vi "Python toolkit.vi"(8 "error in (no error)":errorcluster) -> (0 "error out":errorcluster)   [LabVIEW 2018]
uses:
  Python Toolkit/Python Toolkit.lvclass
  Python Toolkit/Python Toolkit.lvclass/Python Toolkit.ctl
  <vilib>/addons/_JKI Toolkits/Caraya/classes/Assert/Assert Equal Value_Variant.vi
  <vilib>/addons/_JKI Toolkits/Caraya/classes/Assert/Assert Not Error.vi
  <vilib>/addons/_JKI Toolkits/Caraya/classes/Test/Test.lvclass
  <vilib>/addons/_JKI Toolkits/Caraya/classes/Assert/Assert.lvclass
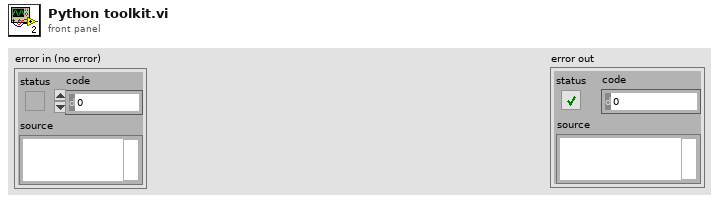
[diagram p1: front panel]
types:
  T1 = cluster{"CCD":string, "S4GUI":string, "S4ICS":string, "TCS":string, "FOCUSER":string, "WSTATION":string, "GENERAL KW":string}
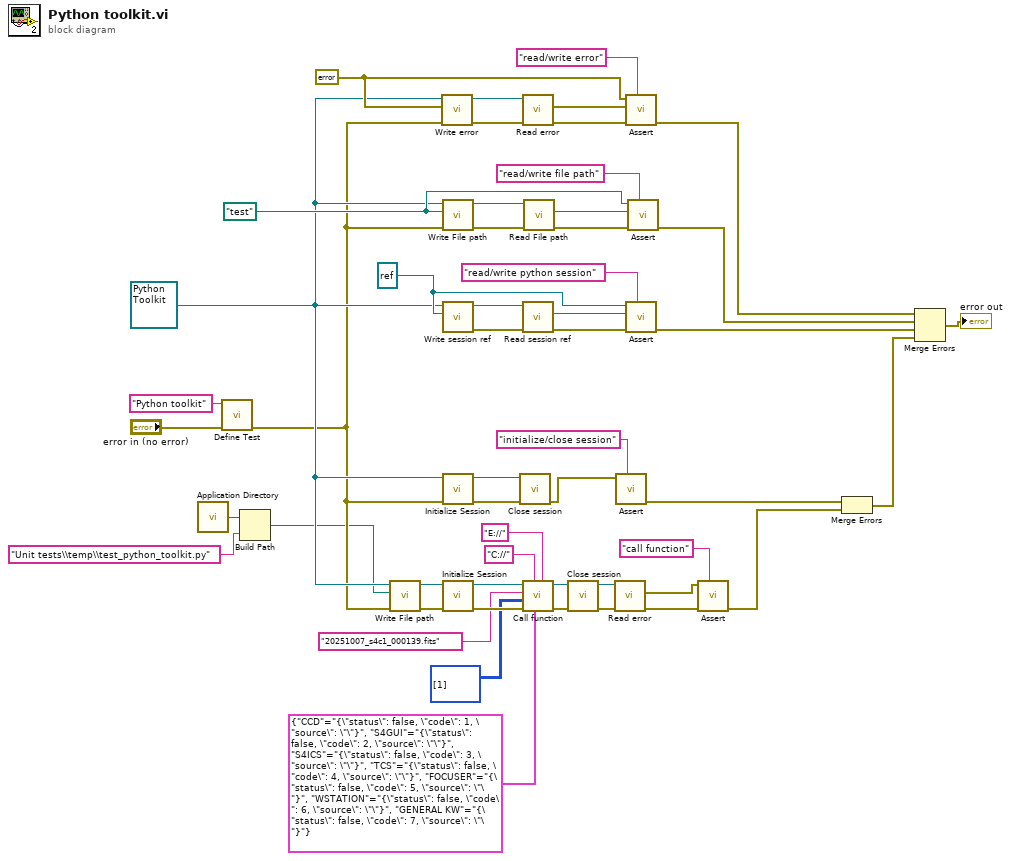
[diagram p0: block diagram]
diagram:
  w29 = refnum<k35> refnum ("session ref")
  w34 = errorcluster {"status"=TRUE, "code"=1, "source"=""} ("error")
  w31 = path "test" ("File path")
  w10 = refnum<class "Python Toolkit.lvclass"> refnum ("Python Toolkit.lvclass")
  n1 = call <vilib>:"Application Directory.vi"() -> ("Application Directory"=w8:path)
  n2 = call <vilib>:"Define Test.vi"("error in (no error)"="error in (no error)", "Label (VI Title)"="Python toolkit") -> ("error out"=w9:errorcluster)  [unwired: 8 in, 1 out]
  n3 = Build Path(base path=w8, name or relative path="Unit tests\\temp\\test_python_toolkit.py") -> (appended path=w6:path)
  n4 = call "Write File path.vi"("error in (no error)"=w9, "File path"=w6, "Python Toolkit in"=w10) -> ("error out"=w12:errorcluster, "Python Toolkit out"=w11:refnum<class "Python Toolkit.lvclass">)  [unwired: 7 in]
  n5 = call "Write error.vi"("error in (no error)"=w9, "error"=w34, "Python Toolkit in"=w10) -> ("error out"=w50:errorcluster, "Python Toolkit out"=w49:refnum<class "Python Toolkit.lvclass">)  [unwired: 7 in]
  n6 = call "Write File path.vi"("error in (no error)"=w9, "File path"=w31, "Python Toolkit in"=w10) -> ("error out"=w47:errorcluster, "Python Toolkit out"=w48:refnum<class "Python Toolkit.lvclass">)  [unwired: 7 in]
  n7 = call-dynamic "Write session ref.vi"("session ref"=w29, "Python Toolkit in"=w10) -> ("error out"=w45:errorcluster, "Python Toolkit out"=w46:refnum<class "Python Toolkit.lvclass">)  [unwired: 8 in]
  n8 = call "Initialize Session.vi"("error in (no error)"=w9, "Python Toolkit in"=w10) -> ("error out"=w25:errorcluster, "Python Toolkit out"=w24:refnum<class "Python Toolkit.lvclass">)  [unwired: 8 in]
  n9 = call "Initialize Session.vi"("error in (no error)"=w12, "Python Toolkit in"=w11) -> ("error out"=w22:errorcluster, "Python Toolkit out"=w21:refnum<class "Python Toolkit.lvclass">)  [unwired: 8 in]
  n10 = call "Close session.vi"("error in (no error)"=w25, "Python Toolkit in"=w24) -> ("error out"=w23:errorcluster)  [unwired: 8 in, 1 out]
  n11 = call "Read error.vi"("error in (no error)"=w50, "Python Toolkit in"=w49) -> ("error out"=w43:errorcluster, "error"=w39:errorcluster)  [unwired: 7 in, 1 out]
  n12 = call-dynamic "Read session ref.vi"("error in (no error)"=w45, "Python Toolkit in"=w46) -> ("error out"=w42:errorcluster, "session ref"=w41:refnum<k35>)  [unwired: 7 in, 1 out]
  n13 = call "Call function.vi"("log file path"="E://", "cluster of jsons"=T1 {"CCD"="{\"status\": false, \"code\": 1, \"source\": \"\"}", "S4GUI"="{\"status\": false, \"code\": 2, \"source\": \"\"}", "S4ICS"="{\"status\": false, \"code\": 3, \"source\": \"\"}", "TCS"="{\"status\": false, \"code\": 4, \"source\": \"\"}", "FOCUSER"="{\"status\": false, \"code\": 5, \"source\": \"\"}", "WSTATION"="{\"status\": false, \"code\": 6, \"source\": \"\"}", "GENERAL KW"="{\"status\": false, \"code\": 7, \"source\": \"\"}"}, "night dir"="C://", "error in (no error)"=w22, "Array"=u16[][] [[1]], "file name"="20251007_s4c1_000139.fits", "Python Toolkit in"=w21) -> ("error out"=w20:errorcluster, "Python Toolkit out"=w19:refnum<class "Python Toolkit.lvclass">)  [unwired: 3 in]
  n14 = call-dynamic "Read File path.vi"("error in (no error)"=w47, "Python Toolkit in"=w48) -> ("error out"=w44:errorcluster, "File path"=w40:path)  [unwired: 7 in, 1 out]
  n15 = call "Close session.vi"("error in (no error)"=w20, "Python Toolkit in"=w19) -> ("error out"=w16:errorcluster, "Python Toolkit out"=w15:refnum<class "Python Toolkit.lvclass">)  [unwired: 8 in]
  n16 = call "Read error.vi"("error in (no error)"=w16, "Python Toolkit in"=w15) -> ("error out"=w14:errorcluster, "error"=w13:errorcluster)  [unwired: 7 in, 1 out]
  n17 = call-poly <vilib>:"Assert.vi"("Label"="initialize/close session" ("Label (VI Title)"), "Not Error?"=w23) -> ("error out"=w28:errorcluster)  [unwired: 8 in, 1 out]
  n18 = call-poly <vilib>:"Assert.vi"("Label"="read/write error" ("Label (VI Title)"), "error in (no error)"=w43, "Actual"=w39, "Expected"=w34) -> ("error out"=w36:errorcluster)  [unwired: 6 in, 1 out]
  n19 = call-poly <vilib>:"Assert.vi"("Label"="read/write python session" ("Label (VI Title)"), "error in (no error)"=w42, "Actual"=w41, "Expected"=w29) -> ("error out"=w38:errorcluster)  [unwired: 6 in, 1 out]
  n20 = call-poly <vilib>:"Assert.vi"("Label"="read/write file path" ("Label (VI Title)"), "error in (no error)"=w44, "Actual"=w40, "Expected"=w31) -> ("error out"=w37:errorcluster)  [unwired: 6 in, 1 out]
  n21 = call-poly <vilib>:"Assert.vi"("Label"="call function" ("Label (VI Title)"), "error in (no error)"=w14, "Not Error?"=w13) -> ("error out"=w18:errorcluster)  [unwired: 7 in, 1 out]
  n22 = Merge Errors(w28, w18) -> (w27:errorcluster)
  n23 = Merge Errors(w36, w37, w38, w27) -> (→"error out":errorcluster)
